vi "initializeDefaultStyle.vi"(8 "error in (no error)":errorcluster, 11 "Title in":refnum<class "Title.lvclass">) -> (0 "error out":errorcluster, 3 "Title out":refnum<class "Title.lvclass">)   [LabVIEW 2020, in "Styles.lvlib" / "Title.lvclass"]
uses:
  Title.lvclass
  D:/Benjamin/Documents/Perso/Code/WC/LabVIEW_NPOI/src/Styles/Style/Style.lvclass
  Alignment--ring.ctl
  Style/Style.lvclass
  Styles.lvlib
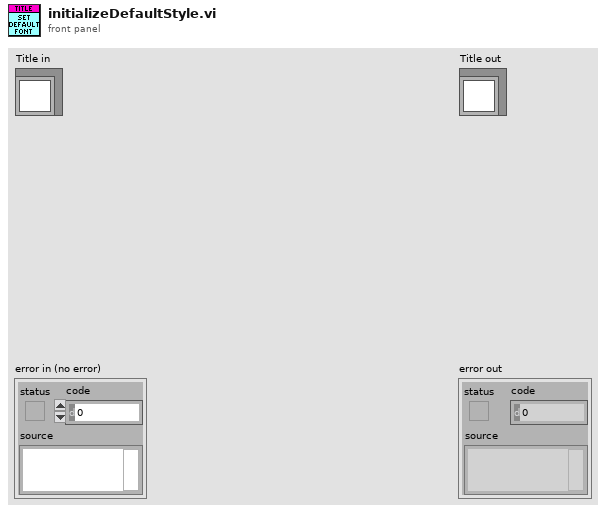
[diagram p1: front panel]
types:
  T1 = typedef "Styles.lvlib/Alignment--ring.ctl" = i32
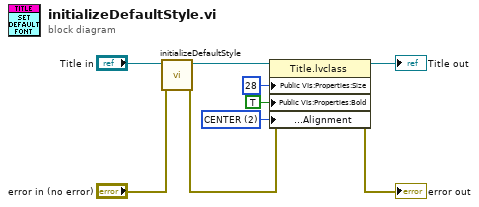
[diagram p0: block diagram]
diagram:
  w1 = T1 2 items=["LEFT"=1, "CENTER"=2, "RIGHT"=3, "BOTH"=4, "MEDIUM_KASHIDA"=5, "DISTRIBUTE"=6, "NUM_TAB"=7, "HIGH_KASHIDA"=8, "LOW_KASHIDA"=9, "THAI_DISTRIBUTE"=10] ("Style:Alignment")
  n1 = call-parent "initializeDefaultStyle.vi"("error in (no error)"="error in (no error)", "Style in"="Title in") -> ("error out"=w5:errorcluster, "Style out"=w9:refnum<class "Title.lvclass">)  [unwired: 8 in]
  n2 = property class="Title.lvclass"(reference=w9, error in=w5, "Public VIs:Properties:Size"=28 ("Style:Size"), "Public VIs:Properties:Bold"=TRUE ("Style:Bold"), "Public VIs:Properties:Alignment"=w1) -> (reference out=→"Title out":refnum<class "Title.lvclass">, error out=→"error out":errorcluster)
